vi "all_subvis.vi"   [LabVIEW 8.6]
uses:
  Controls/lxw_alignment.ctl
  Controls/lxw_boolean.ctl
  Controls/lxw_border_style.ctl
  Controls/lxw_chart_axis_label_position.ctl
  Controls/lxw_chart_axis_type.ctl
  Controls/lxw_chart_legend_position.ctl
  Controls/lxw_chart_marker_type.ctl
  Controls/lxw_chart_type.ctl
  Controls/lxw_defined_colors.ctl
  Controls/lxw_error.ctl
  Controls/lxw_filter_criteria.ctl
  Controls/lxw_filter_operator.ctl
  Controls/lxw_filter_rule.ctl
  Controls/lxw_pattern_type.ctl
  Controls/style_id.ctl
types:
  T1 = typedef "style_id.ctl" = u16
  T2 = typedef "lxw_pattern_type.ctl" = u8
  T3 = typedef "lxw_filter_rule.ctl" = cluster{"criteria":T4, "value_string":string, "value":dbl}
  T4 = typedef "lxw_filter_criteria.ctl" = u32
  T5 = typedef "lxw_filter_operator.ctl" = u8
  T6 = typedef "lxw_error.ctl" = u32
  T7 = typedef "lxw_defined_colors.ctl" = u32
  T8 = typedef "lxw_chart_type.ctl" = u8
  T9 = typedef "lxw_chart_marker_type.ctl" = u8
  T10 = typedef "lxw_chart_legend_position.ctl" = u8
  T11 = typedef "lxw_chart_axis_type.ctl" = u8
  T12 = typedef "lxw_chart_axis_label_position.ctl" = u8
  T13 = typedef "lxw_border_style.ctl" = u8
  T14 = typedef "lxw_boolean.ctl" = u8
  T15 = typedef "lxw_alignment.ctl" = u8
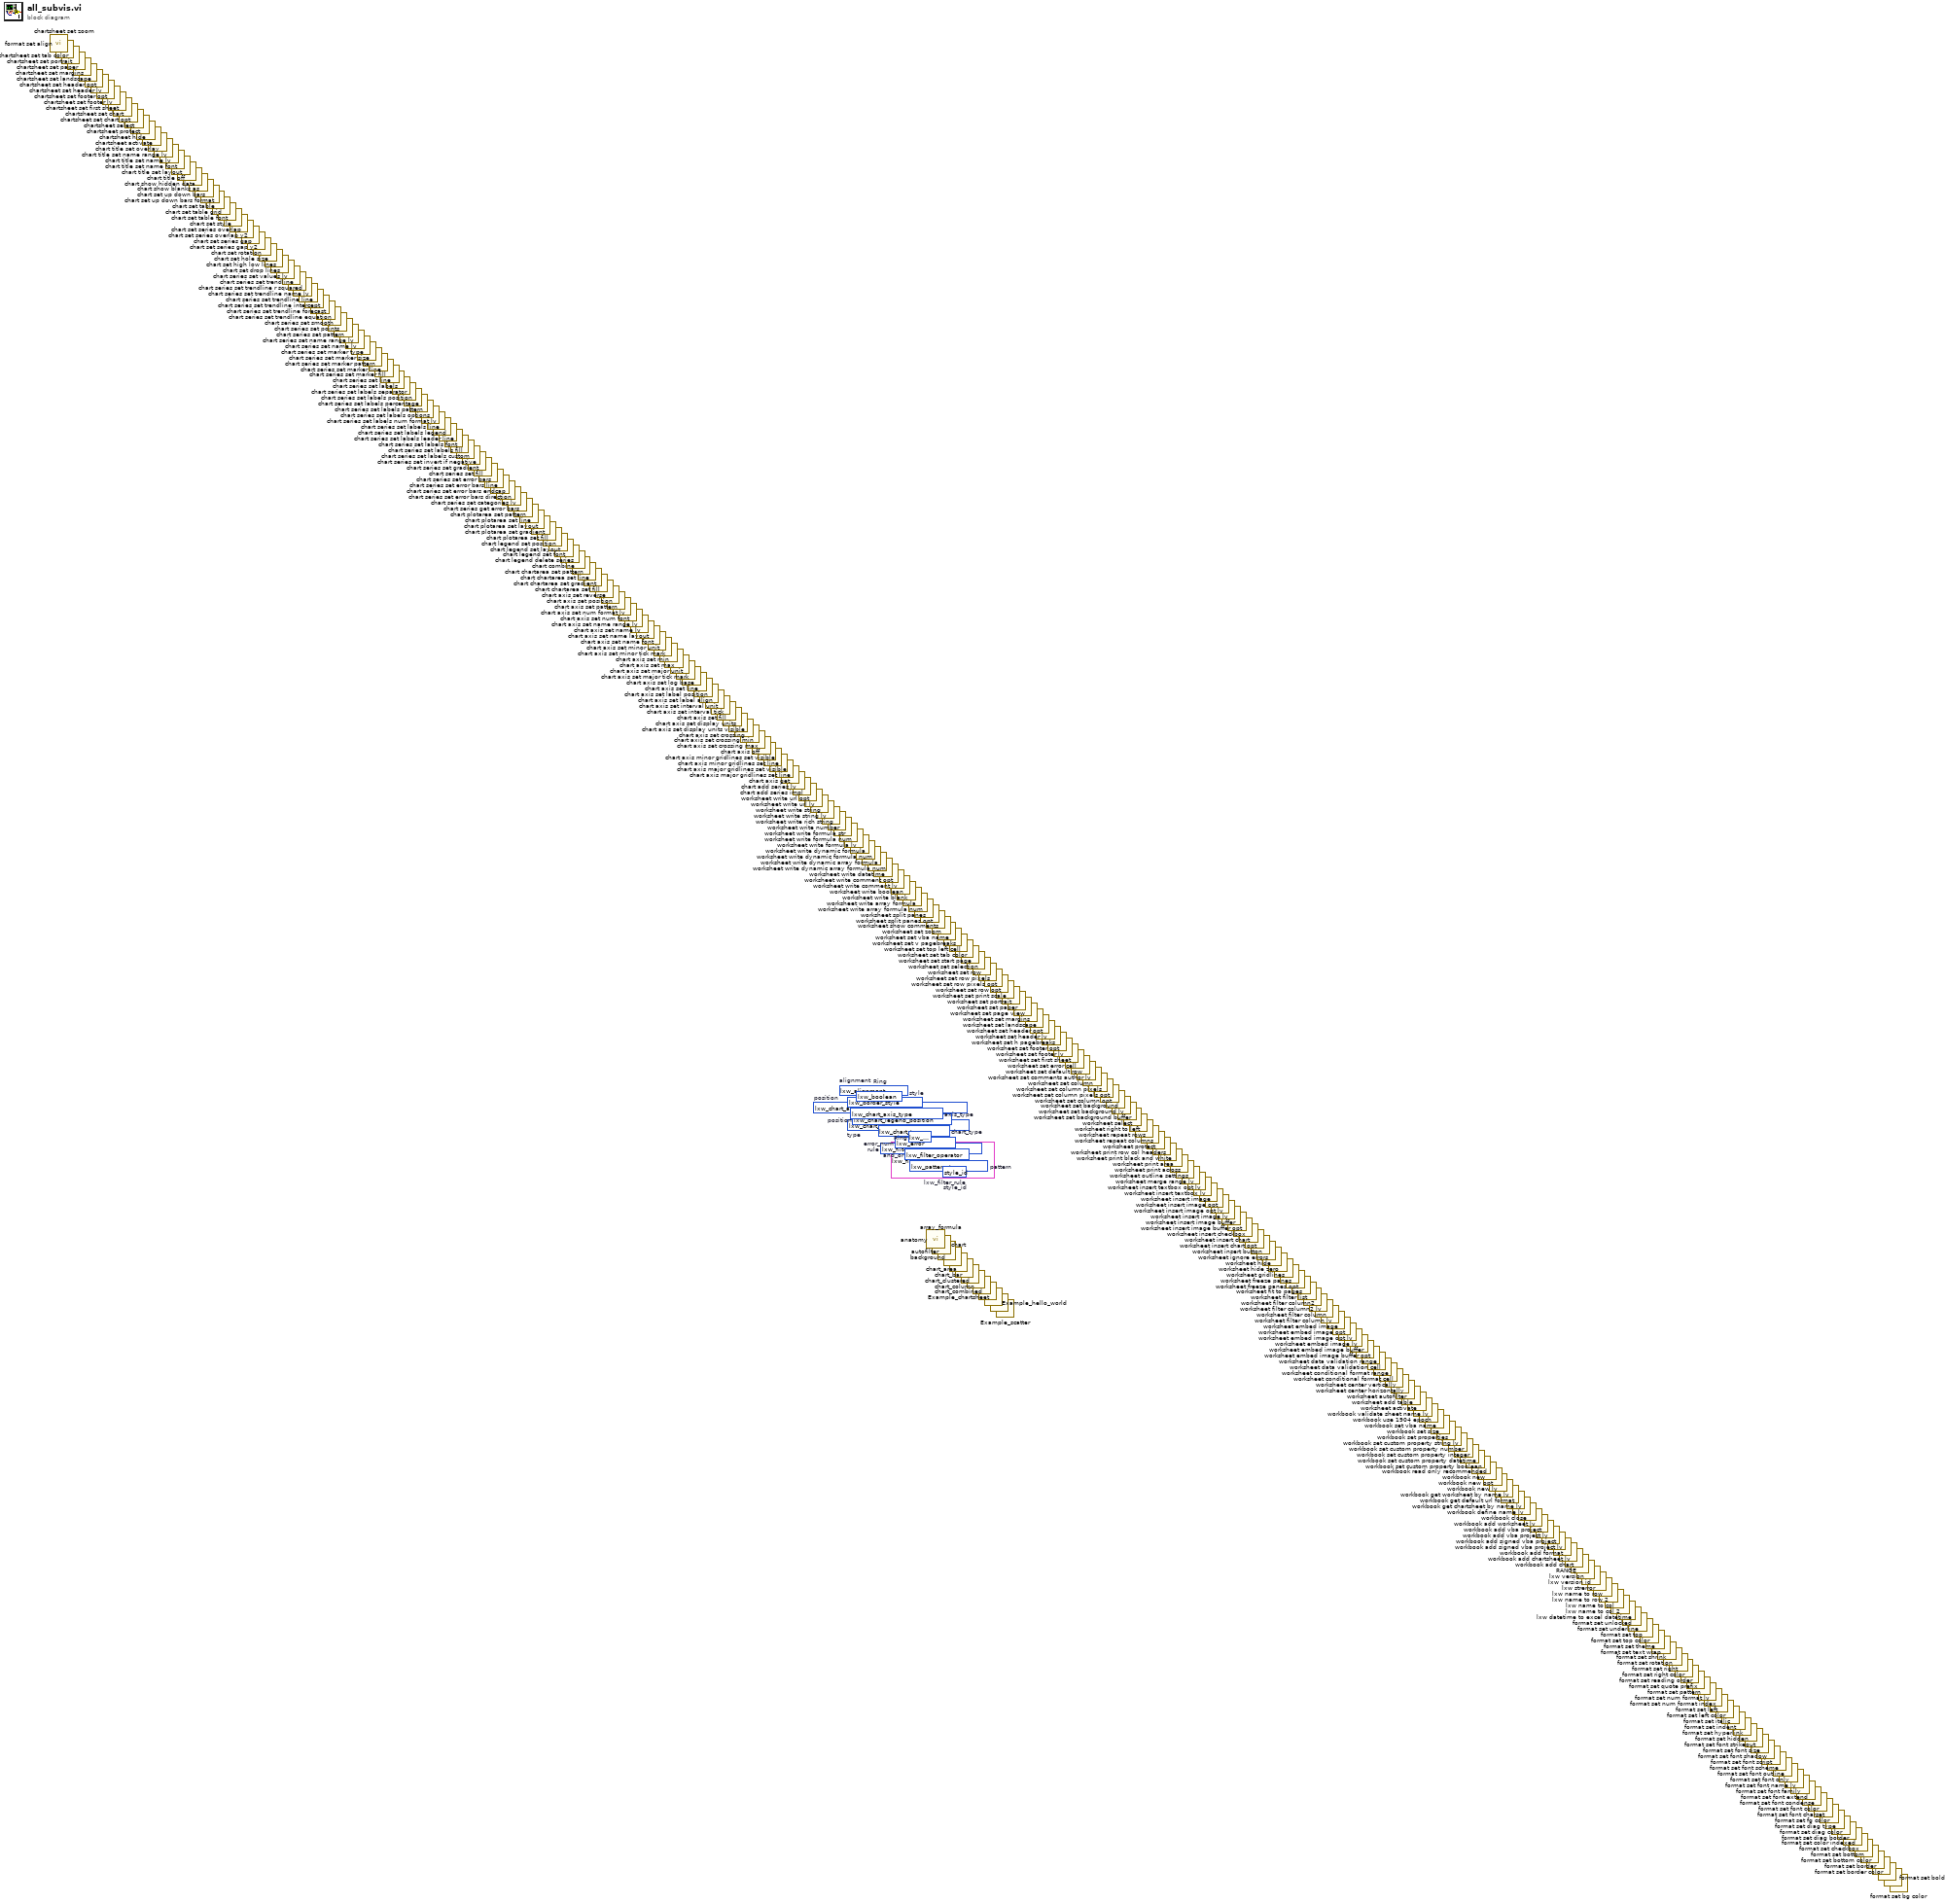
[diagram p0: block diagram]
diagram:
  (unwired) T1 ? items=["Style_1", "Style_2", "Style_3", "Style_4", "Style_5", "Style_6", "Style_7", "Style_8", "Style_9", "Style_10", "Style_11", "Style_12", "Style_13", "Style_14", "Style_15", "Style_16", "Style_17", "Style_18", "Style_19", "Style_20", "Style_21", "Style_22", "Style_23", "Style_24", "Style_25", "Style_26", "Style_27", "Style_28", "Style_29", "Style_30", "Style_31", "Style_32", "Style_33", "Style_34", "Style_35", "Style_36", "Style_37", "Style_38", "Style_39", "Style_40", "Style_41", "Style_42", "Style_43", "Style_44", "Style_45", "Style_46", "Style_47", "Style_48"]  # style_id
  (unwired) T2 ? items=["LXW_PATTERN_NONE", "LXW_PATTERN_SOLID", "LXW_PATTERN_MEDIUM_GRAY", "LXW_PATTERN_DARK_GRAY", "LXW_PATTERN_LIGHT_GRAY"]  # pattern
  (unwired) T3 ?  # lxw_filter_rule
  (unwired) T5 ? items=["LXW_FILTER_AND", "LXW_FILTER_OR"]  # and_or
  (unwired) T4 ? items=["LXW_FILTER_CRITERIA_NONE", "LXW_FILTER_CRITERIA_EQUAL_TO", "LXW_FILTER_CRITERIA_NOT_EQUAL_TO", "LXW_FILTER_CRITERIA_GREATER_THAN", "LXW_FILTER_CRITERIA_LESS_THAN", "LXW_FILTER_CRITERIA_GREATER_THAN_OR_EQUAL_TO", "LXW_FILTER_CRITERIA_LESS_THAN_OR_EQUAL_TO", "LXW_FILTER_CRITERIA_BLANKS", "LXW_FILTER_CRITERIA_NON_BLANKS"]  # rule
  (unwired) T6 ? items=["LXW_NO_ERROR", "LXW_ERROR_MEMORY_MALLOC_FAILED", "LXW_ERROR_CREATING_XLSX_FILE", "LXW_ERROR_CREATING_TMPFILE", "LXW_ERROR_READING_TMPFILE", "LXW_ERROR_ZIP_FILE_OPERATION", "LXW_ERROR_ZIP_PARAMETER_ERROR", "LXW_ERROR_ZIP_BAD_ZIP_FILE", "LXW_ERROR_ZIP_INTERNAL_ERROR", "LXW_ERROR_ZIP_FILE_ADD", "LXW_ERROR_ZIP_CLOSE", "LXW_ERROR_FEATURE_NOT_SUPPORTED", "LXW_ERROR_NULL_PARAMETER_IGNORED", "LXW_ERROR_PARAMETER_VALIDATION", "LXW_ERROR_WORKSHEET_INDEX_OUT_OF_RANGE"]  # error_num
  (unwired) T7 ? items=["LXW_COLOR_BLACK", "LXW_COLOR_BLUE", "LXW_COLOR_BROWN", "LXW_COLOR_CYAN", "LXW_COLOR_GRAY", "LXW_COLOR_GREEN", "LXW_COLOR_LIME", "LXW_COLOR_MAGENTA", "LXW_COLOR_NAVY", "LXW_COLOR_ORANGE", "LXW_COLOR_PURPLE", "LXW_COLOR_RED", "LXW_COLOR_SILVER", "LXW_COLOR_WHITE", "LXW_COLOR_YELLOW"]  # Ring
  (unwired) T8 ? items=["LXW_CHART_NONE", "LXW_CHART_AREA", "LXW_CHART_AREA_STACKED", "LXW_CHART_AREA_STACKED_PERCENT", "LXW_CHART_BAR", "LXW_CHART_BAR_STACKED", "LXW_CHART_BAR_STACKED_PERCENT", "LXW_CHART_COLUMN", "LXW_CHART_COLUMN_STACKED", "LXW_CHART_COLUMN_STACKED_PERCENT", "LXW_CHART_DOUGHNUT", "LXW_CHART_LINE", "LXW_CHART_LINE_STACKED", "LXW_CHART_LINE_STACKED_PERCENT", "LXW_CHART_PIE", "LXW_CHART_SCATTER", "LXW_CHART_SCATTER_STRAIGHT", "LXW_CHART_SCATTER_STRAIGHT_WITH_MARKERS", "LXW_CHART_SCATTER_SMOOTH", "LXW_CHART_SCATTER_SMOOTH_WITH_MARKERS", "LXW_CHART_RADAR", "LXW_CHART_RADAR_WITH_MARKERS", "LXW_CHART_RADAR_FILLED", "LXW_CHART_STOCK"]  # chart_type
  (unwired) T9 ? items=["LXW_CHART_MARKER_AUTOMATIC", "LXW_CHART_MARKER_NONE", "LXW_CHART_MARKER_SQUARE", "LXW_CHART_MARKER_DIAMOND", "LXW_CHART_MARKER_TRIANGLE", "LXW_CHART_MARKER_X", "LXW_CHART_MARKER_STAR", "LXW_CHART_MARKER_SHORT_DASH", "LXW_CHART_MARKER_LONG_DASH", "LXW_CHART_MARKER_CIRCLE", "LXW_CHART_MARKER_PLUS"]  # type
  (unwired) T10 ? items=["LXW_CHART_LEGEND_NONE", "LXW_CHART_LEGEND_RIGHT", "LXW_CHART_LEGEND_LEFT", "LXW_CHART_LEGEND_TOP", "LXW_CHART_LEGEND_BOTTOM", "LXW_CHART_LEGEND_TOP_RIGHT", "LXW_CHART_LEGEND_OVERLAY_RIGHT", "LXW_CHART_LEGEND_OVERLAY_LEFT"]  # position
  (unwired) T11 ? items=["LXW_CHART_AXIS_TYPE_X", "LXW_CHART_AXIS_TYPE_Y", "LXW_CHART_AXIS_TYPE_X2", "LXW_CHART_AXIS_TYPE_Y2"]  # axis_type
  (unwired) T12 ? items=["LXW_CHART_AXIS_LABEL_POSITION_NEXT_TO", "LXW_CHART_AXIS_LABEL_POSITION_HIGH", "LXW_CHART_AXIS_LABEL_POSITION_LOW", "LXW_CHART_AXIS_LABEL_POSITION_NONE"]  # position
  (unwired) T13 ? items=["LXW_BORDER_NONE", "LXW_BORDER_THIN", "LXW_BORDER_MEDIUM", "LXW_BORDER_DASHED", "LXW_BORDER_DOTTED", "LXW_BORDER_THICK", "LXW_BORDER_DOUBLE", "LXW_BORDER_HAIR"]  # style
  (unwired) T14 ? items=["LXW_FALSE", "LXW_TRUE", "LXW_EXPLICIT_FALSE"]  # Ring
  (unwired) T15 ? items=["LXW_ALIGN_NONE", "LXW_ALIGN_LEFT", "LXW_ALIGN_CENTER", "LXW_ALIGN_RIGHT", "LXW_ALIGN_FILL", "LXW_ALIGN_JUSTIFY", "LXW_ALIGN_CENTER_ACROSS", "LXW_ALIGN_DISTRIBUTED", "LXW_ALIGN_VERTICAL_TOP", "LXW_ALIGN_VERTICAL_BOTTOM", "LXW_ALIGN_VERTICAL_CENTER", "LXW_ALIGN_VERTICAL_JUSTIFY", "LXW_ALIGN_VERTICAL_DISTRIBUTED"]  # alignment
  n1 = call "format set align.vi"() -> ()  [unwired: 11 in, 1 out]
  n2 = call "chartsheet set zoom.vi"() -> ()  [unwired: 11 in, 1 out]
  n3 = call "chartsheet set tab color.vi"() -> ()  [unwired: 11 in, 1 out]
  n4 = call "chartsheet set portrait.vi"() -> ()  [unwired: 11 in, 1 out]
  n5 = call "chartsheet set paper.vi"() -> ()  [unwired: 11 in, 1 out]
  n6 = call "chartsheet set margins.vi"() -> ()  [unwired: 11 in, 1 out]
  n7 = call "chartsheet set landscape.vi"() -> ()  [unwired: 11 in, 1 out]
  n8 = call "chartsheet set header opt.vi"() -> ()  [unwired: 9 in, 3 out]
  n9 = call "chartsheet set header lv.vi"() -> ()  [unwired: 10 in, 2 out]
  n10 = call "chartsheet set footer opt.vi"() -> ()  [unwired: 9 in, 3 out]
  n11 = call "chartsheet set footer lv.vi"() -> ()  [unwired: 10 in, 2 out]
  n12 = call "chartsheet set first sheet.vi"() -> ()  [unwired: 11 in, 1 out]
  n13 = call "chartsheet set chart.vi"() -> ()  [unwired: 10 in, 2 out]
  n14 = call "chartsheet set chart opt.vi"() -> ()  [unwired: 9 in, 3 out]
  n15 = call "chartsheet select.vi"() -> ()  [unwired: 11 in, 1 out]
  n16 = call "chartsheet protect.vi"() -> ()  [unwired: 10 in, 2 out]
  n17 = call "chartsheet hide.vi"() -> ()  [unwired: 11 in, 1 out]
  n18 = call "chartsheet activate.vi"() -> ()  [unwired: 11 in, 1 out]
  n19 = call "chart title set overlay.vi"() -> ()  [unwired: 11 in, 1 out]
  n20 = call "chart title set name range lv.vi"() -> ()  [unwired: 11 in, 1 out]
  n21 = call "chart title set name lv.vi"() -> ()  [unwired: 11 in, 1 out]
  n22 = call "chart title set name font.vi"() -> ()  [unwired: 10 in, 2 out]
  n23 = call "chart title set layout.vi"() -> ()  [unwired: 10 in, 2 out]
  n24 = call "chart title off.vi"() -> ()  [unwired: 11 in, 1 out]
  n25 = call "chart show hidden data.vi"() -> ()  [unwired: 11 in, 1 out]
  n26 = call "chart show blanks as.vi"() -> ()  [unwired: 11 in, 1 out]
  n27 = call "chart set up down bars.vi"() -> ()  [unwired: 11 in, 1 out]
  n28 = call "chart set up down bars format.vi"() -> ()  [unwired: 11 in, 5 out]
  n29 = call "chart set table.vi"() -> ()  [unwired: 11 in, 1 out]
  n30 = call "chart set table grid.vi"() -> ()  [unwired: 11 in, 1 out]
  n31 = call "chart set table font.vi"() -> ()  [unwired: 10 in, 2 out]
  n32 = call "chart set style.vi"() -> ()  [unwired: 11 in, 1 out]
  n33 = call "chart set series overlap.vi"() -> ()  [unwired: 11 in, 1 out]
  n34 = call "chart set series overlap y2.vi"() -> ()  [unwired: 11 in, 1 out]
  n35 = call "chart set series gap.vi"() -> ()  [unwired: 11 in, 1 out]
  n36 = call "chart set series gap y2.vi"() -> ()  [unwired: 11 in, 1 out]
  n37 = call "chart set rotation.vi"() -> ()  [unwired: 11 in, 1 out]
  n38 = call "chart set hole size.vi"() -> ()  [unwired: 11 in, 1 out]
  n39 = call "chart set high low lines.vi"() -> ()  [unwired: 10 in, 2 out]
  n40 = call "chart set drop lines.vi"() -> ()  [unwired: 10 in, 2 out]
  n41 = call "chart series set values lv.vi"() -> ()  [unwired: 11 in, 1 out]
  n42 = call "chart series set trendline.vi"() -> ()  [unwired: 11 in, 1 out]
  n43 = call "chart series set trendline r squared.vi"() -> ()  [unwired: 11 in, 1 out]
  n44 = call "chart series set trendline name lv.vi"() -> ()  [unwired: 11 in, 1 out]
  n45 = call "chart series set trendline line.vi"() -> ()  [unwired: 10 in, 2 out]
  n46 = call "chart series set trendline intercept.vi"() -> ()  [unwired: 11 in, 1 out]
  n47 = call "chart series set trendline forecast.vi"() -> ()  [unwired: 11 in, 1 out]
  n48 = call "chart series set trendline equation.vi"() -> ()  [unwired: 11 in, 1 out]
  n49 = call "chart series set smooth.vi"() -> ()  [unwired: 11 in, 1 out]
  n50 = call "chart series set points.vi"() -> ()  [unwired: 10 in, 2 out]
  n51 = call "chart series set pattern.vi"() -> ()  [unwired: 10 in, 2 out]
  n52 = call "chart series set name range lv.vi"() -> ()  [unwired: 11 in, 1 out]
  n53 = call "chart series set name lv.vi"() -> ()  [unwired: 11 in, 1 out]
  n54 = call "chart series set marker type.vi"() -> ()  [unwired: 11 in, 1 out]
  n55 = call "chart series set marker size.vi"() -> ()  [unwired: 11 in, 1 out]
  n56 = call "chart series set marker pattern.vi"() -> ()  [unwired: 10 in, 2 out]
  n57 = call "chart series set marker line.vi"() -> ()  [unwired: 10 in, 2 out]
  n58 = call "chart series set marker fill.vi"() -> ()  [unwired: 10 in, 2 out]
  n59 = call "chart series set line.vi"() -> ()  [unwired: 10 in, 2 out]
  n60 = call "chart series set labels.vi"() -> ()  [unwired: 11 in, 1 out]
  n61 = call "chart series set labels separator.vi"() -> ()  [unwired: 11 in, 1 out]
  n62 = call "chart series set labels position.vi"() -> ()  [unwired: 11 in, 1 out]
  n63 = call "chart series set labels percentage.vi"() -> ()  [unwired: 11 in, 1 out]
  n64 = call "chart series set labels pattern.vi"() -> ()  [unwired: 10 in, 2 out]
  n65 = call "chart series set labels options.vi"() -> ()  [unwired: 11 in, 1 out]
  n66 = call "chart series set labels num format lv.vi"() -> ()  [unwired: 11 in, 1 out]
  n67 = call "chart series set labels line.vi"() -> ()  [unwired: 10 in, 2 out]
  n68 = call "chart series set labels legend.vi"() -> ()  [unwired: 11 in, 1 out]
  n69 = call "chart series set labels leader line.vi"() -> ()  [unwired: 11 in, 1 out]
  n70 = call "chart series set labels font.vi"() -> ()  [unwired: 10 in, 2 out]
  n71 = call "chart series set labels fill.vi"() -> ()  [unwired: 10 in, 2 out]
  n72 = call "chart series set labels custom.vi"() -> ()  [unwired: 10 in, 2 out]
  n73 = call "chart series set invert if negative.vi"() -> ()  [unwired: 11 in, 1 out]
  n74 = call "chart series set gradient.vi"() -> ()  [unwired: 10 in, 2 out]
  n75 = call "chart series set fill.vi"() -> ()  [unwired: 10 in, 2 out]
  n76 = call "chart series set error bars.vi"() -> ()  [unwired: 11 in, 1 out]
  n77 = call "chart series set error bars line.vi"() -> ()  [unwired: 10 in, 2 out]
  n78 = call "chart series set error bars endcap.vi"() -> ()  [unwired: 11 in, 1 out]
  n79 = call "chart series set error bars direction.vi"() -> ()  [unwired: 11 in, 1 out]
  n80 = call "chart series set categories lv.vi"() -> ()  [unwired: 11 in, 1 out]
  n81 = call "chart series get error bars.vi"() -> ()  [unwired: 10 in, 2 out]
  n82 = call "chart plotarea set pattern.vi"() -> ()  [unwired: 10 in, 2 out]
  n83 = call "chart plotarea set line.vi"() -> ()  [unwired: 10 in, 2 out]
  n84 = call "chart plotarea set layout.vi"() -> ()  [unwired: 10 in, 2 out]
  n85 = call "chart plotarea set gradient.vi"() -> ()  [unwired: 10 in, 2 out]
  n86 = call "chart plotarea set fill.vi"() -> ()  [unwired: 10 in, 2 out]
  n87 = call "chart legend set position.vi"() -> ()  [unwired: 11 in, 1 out]
  n88 = call "chart legend set layout.vi"() -> ()  [unwired: 10 in, 2 out]
  n89 = call "chart legend set font.vi"() -> ()  [unwired: 10 in, 2 out]
  n90 = call "chart legend delete series.vi"() -> ()  [unwired: 10 in, 2 out]
  n91 = call "chart combine.vi"() -> ()  [unwired: 11 in, 1 out]
  n92 = call "chart chartarea set pattern.vi"() -> ()  [unwired: 10 in, 2 out]
  n93 = call "chart chartarea set line.vi"() -> ()  [unwired: 10 in, 2 out]
  n94 = call "chart chartarea set gradient.vi"() -> ()  [unwired: 10 in, 2 out]
  n95 = call "chart chartarea set fill.vi"() -> ()  [unwired: 10 in, 2 out]
  n96 = call "chart axis set reverse.vi"() -> ()  [unwired: 11 in, 1 out]
  n97 = call "chart axis set position.vi"() -> ()  [unwired: 11 in, 1 out]
  n98 = call "chart axis set pattern.vi"() -> ()  [unwired: 10 in, 2 out]
  n99 = call "chart axis set num format lv.vi"() -> ()  [unwired: 11 in, 1 out]
  n100 = call "chart axis set num font.vi"() -> ()  [unwired: 10 in, 2 out]
  n101 = call "chart axis set name range lv.vi"() -> ()  [unwired: 11 in, 1 out]
  n102 = call "chart axis set name lv.vi"() -> ()  [unwired: 11 in, 1 out]
  n103 = call "chart axis set name layout.vi"() -> ()  [unwired: 10 in, 2 out]
  n104 = call "chart axis set name font.vi"() -> ()  [unwired: 10 in, 2 out]
  n105 = call "chart axis set minor unit.vi"() -> ()  [unwired: 11 in, 1 out]
  n106 = call "chart axis set minor tick mark.vi"() -> ()  [unwired: 11 in, 1 out]
  n107 = call "chart axis set min.vi"() -> ()  [unwired: 11 in, 1 out]
  n108 = call "chart axis set max.vi"() -> ()  [unwired: 11 in, 1 out]
  n109 = call "chart axis set major unit.vi"() -> ()  [unwired: 11 in, 1 out]
  n110 = call "chart axis set major tick mark.vi"() -> ()  [unwired: 11 in, 1 out]
  n111 = call "chart axis set log base.vi"() -> ()  [unwired: 11 in, 1 out]
  n112 = call "chart axis set line.vi"() -> ()  [unwired: 10 in, 2 out]
  n113 = call "chart axis set label position.vi"() -> ()  [unwired: 11 in, 1 out]
  n114 = call "chart axis set label align.vi"() -> ()  [unwired: 11 in, 1 out]
  n115 = call "chart axis set interval unit.vi"() -> ()  [unwired: 11 in, 1 out]
  n116 = call "chart axis set interval tick.vi"() -> ()  [unwired: 11 in, 1 out]
  n117 = call "chart axis set fill.vi"() -> ()  [unwired: 10 in, 2 out]
  n118 = call "chart axis set display units.vi"() -> ()  [unwired: 11 in, 1 out]
  n119 = call "chart axis set display units visible.vi"() -> ()  [unwired: 11 in, 1 out]
  n120 = call "chart axis set crossing.vi"() -> ()  [unwired: 11 in, 1 out]
  n121 = call "chart axis set crossing min.vi"() -> ()  [unwired: 11 in, 1 out]
  n122 = call "chart axis set crossing max.vi"() -> ()  [unwired: 11 in, 1 out]
  n123 = call "chart axis off.vi"() -> ()  [unwired: 11 in, 1 out]
  n124 = call "chart axis minor gridlines set visible.vi"() -> ()  [unwired: 11 in, 1 out]
  n125 = call "chart axis minor gridlines set line.vi"() -> ()  [unwired: 10 in, 2 out]
  n126 = call "chart axis major gridlines set visible.vi"() -> ()  [unwired: 11 in, 1 out]
  n127 = call "chart axis major gridlines set line.vi"() -> ()  [unwired: 10 in, 2 out]
  n128 = call "chart axis get.vi"() -> ()  [unwired: 10 in, 2 out]
  n129 = call "chart add series lv.vi"() -> ()  [unwired: 10 in, 2 out]
  n130 = call "chart add series impl.vi"() -> ()  [unwired: 10 in, 2 out]
  n131 = call "worksheet write url opt.vi"() -> ()  [unwired: 10 in, 2 out]
  n132 = call "worksheet write url lv.vi"() -> ()  [unwired: 10 in, 2 out]
  n133 = call "worksheet write string.vi"() -> ()  [unwired: 10 in, 2 out]
  n134 = call "worksheet write string lv.vi"() -> ()  [unwired: 10 in, 2 out]
  n135 = call "worksheet write rich string.vi"() -> ()  [unwired: 10 in, 2 out]
  n136 = call "worksheet write number.vi"() -> ()  [unwired: 10 in, 2 out]
  n137 = call "worksheet write formula str.vi"() -> ()  [unwired: 10 in, 2 out]
  n138 = call "worksheet write formula num.vi"() -> ()  [unwired: 10 in, 2 out]
  n139 = call "worksheet write formula lv.vi"() -> ()  [unwired: 10 in, 2 out]
  n140 = call "worksheet write dynamic formula.vi"() -> ()  [unwired: 10 in, 2 out]
  n141 = call "worksheet write dynamic formula num.vi"() -> ()  [unwired: 10 in, 2 out]
  n142 = call "worksheet write dynamic array formula.vi"() -> ()  [unwired: 10 in, 2 out]
  n143 = call "worksheet write dynamic array formula num.vi"() -> ()  [unwired: 14 in, 2 out]
  n144 = call "worksheet write datetime.vi"() -> ()  [unwired: 9 in, 3 out]
  n145 = call "worksheet write comment opt.vi"() -> ()  [unwired: 10 in, 2 out]
  n146 = call "worksheet write comment lv.vi"() -> ()  [unwired: 10 in, 2 out]
  n147 = call "worksheet write boolean.vi"() -> ()  [unwired: 10 in, 2 out]
  n148 = call "worksheet write blank.vi"() -> ()  [unwired: 10 in, 2 out]
  n149 = call "worksheet write array formula.vi"() -> ()  [unwired: 10 in, 2 out]
  n150 = call "worksheet write array formula num.vi"() -> ()  [unwired: 14 in, 2 out]
  n151 = call "worksheet split panes.vi"() -> ()  [unwired: 11 in, 1 out]
  n152 = call "worksheet split panes opt.vi"() -> ()  [unwired: 11 in, 1 out]
  n153 = call "anatomy.vi"() -> ()  [unwired: 12 in]
  n154 = call "worksheet show comments.vi"() -> ()  [unwired: 11 in, 1 out]
  n155 = call "array_formula.vi"() -> ()  [unwired: 12 in]
  n156 = call "worksheet set zoom.vi"() -> ()  [unwired: 11 in, 1 out]
  n157 = call "autofilter.vi"() -> ()  [unwired: 12 in]
  n158 = call "worksheet set vba name.vi"() -> ()  [unwired: 10 in, 2 out]
  n159 = call "background.vi"() -> ()  [unwired: 12 in]
  n160 = call "worksheet set v pagebreaks.vi"() -> ()  [unwired: 10 in, 2 out]
  n161 = call "chart.vi"() -> ()  [unwired: 12 in]
  n162 = call "worksheet set top left cell.vi"() -> ()  [unwired: 11 in, 1 out]
  n163 = call "chart_area.vi"() -> ()  [unwired: 12 in]
  n164 = call "worksheet set tab color.vi"() -> ()  [unwired: 11 in, 1 out]
  n165 = call "chart_bar.vi"() -> ()  [unwired: 12 in]
  n166 = call "worksheet set start page.vi"() -> ()  [unwired: 11 in, 1 out]
  n167 = call "chart_clustered.vi"() -> ()  [unwired: 12 in]
  n168 = call "worksheet set selection.vi"() -> ()  [unwired: 10 in, 2 out]
  n169 = call "chart_column.vi"() -> ()  [unwired: 12 in]
  n170 = call "worksheet set row.vi"() -> ()  [unwired: 10 in, 2 out]
  n171 = call "chart_combined.vi"() -> ()  [unwired: 12 in]
  n172 = call "worksheet set row pixels.vi"() -> ()  [unwired: 10 in, 2 out]
  n173 = call "Example_chartsheet.vi"() -> ()  [unwired: 12 in]
  n174 = call "worksheet set row pixels opt.vi"() -> ()  [unwired: 9 in, 3 out]
  n175 = call "Example_hello_world.vi"() -> ()  [unwired: 12 in]
  n176 = call "worksheet set row opt.vi"() -> ()  [unwired: 9 in, 3 out]
  n177 = call "Example_scatter.vi"() -> ()  [unwired: 12 in]
  n178 = call "worksheet set print scale.vi"() -> ()  [unwired: 11 in, 1 out]
  n179 = call "worksheet set portrait.vi"() -> ()  [unwired: 11 in, 1 out]
  n180 = call "worksheet set paper.vi"() -> ()  [unwired: 11 in, 1 out]
  n181 = call "worksheet set page view.vi"() -> ()  [unwired: 11 in, 1 out]
  n182 = call "worksheet set margins.vi"() -> ()  [unwired: 11 in, 1 out]
  n183 = call "worksheet set landscape.vi"() -> ()  [unwired: 11 in, 1 out]
  n184 = call "worksheet set header opt.vi"() -> ()  [unwired: 9 in, 3 out]
  n185 = call "worksheet set header lv.vi"() -> ()  [unwired: 10 in, 2 out]
  n186 = call "worksheet set h pagebreaks.vi"() -> ()  [unwired: 10 in, 2 out]
  n187 = call "worksheet set footer opt.vi"() -> ()  [unwired: 9 in, 3 out]
  n188 = call "worksheet set footer lv.vi"() -> ()  [unwired: 10 in, 2 out]
  n189 = call "worksheet set first sheet.vi"() -> ()  [unwired: 11 in, 1 out]
  n190 = call "worksheet set error cell.vi"() -> ()  [unwired: 11 in, 1 out]
  n191 = call "worksheet set default row.vi"() -> ()  [unwired: 11 in, 1 out]
  n192 = call "worksheet set comments author lv.vi"() -> ()  [unwired: 11 in, 1 out]
  n193 = call "worksheet set column.vi"() -> ()  [unwired: 10 in, 2 out]
  n194 = call "worksheet set column pixels.vi"() -> ()  [unwired: 10 in, 2 out]
  n195 = call "worksheet set column pixels opt.vi"() -> ()  [unwired: 9 in, 3 out]
  n196 = call "worksheet set column opt.vi"() -> ()  [unwired: 9 in, 3 out]
  n197 = call "worksheet set background.vi"() -> ()  [unwired: 10 in, 2 out]
  n198 = call "worksheet set background lv.vi"() -> ()  [unwired: 10 in, 2 out]
  n199 = call "worksheet set background buffer.vi"() -> ()  [unwired: 10 in, 2 out]
  n200 = call "worksheet select.vi"() -> ()  [unwired: 11 in, 1 out]
  n201 = call "worksheet right to left.vi"() -> ()  [unwired: 11 in, 1 out]
  n202 = call "worksheet repeat rows.vi"() -> ()  [unwired: 10 in, 2 out]
  n203 = call "worksheet repeat columns.vi"() -> ()  [unwired: 10 in, 2 out]
  n204 = call "worksheet protect.vi"() -> ()  [unwired: 10 in, 2 out]
  n205 = call "worksheet print row col headers.vi"() -> ()  [unwired: 11 in, 1 out]
  n206 = call "worksheet print black and white.vi"() -> ()  [unwired: 11 in, 1 out]
  n207 = call "worksheet print area.vi"() -> ()  [unwired: 10 in, 2 out]
  n208 = call "worksheet print across.vi"() -> ()  [unwired: 11 in, 1 out]
  n209 = call "worksheet outline settings.vi"() -> ()  [unwired: 11 in, 1 out]
  n210 = call "worksheet merge range lv.vi"() -> ()  [unwired: 10 in, 2 out]
  n211 = call "worksheet insert textbox opt lv.vi"() -> ()  [unwired: 9 in, 3 out]
  n212 = call "worksheet insert textbox lv.vi"() -> ()  [unwired: 10 in, 2 out]
  n213 = call "worksheet insert image.vi"() -> ()  [unwired: 10 in, 2 out]
  n214 = call "worksheet insert image opt.vi"() -> ()  [unwired: 9 in, 3 out]
  n215 = call "worksheet insert image opt lv.vi"() -> ()  [unwired: 9 in, 3 out]
  n216 = call "worksheet insert image lv.vi"() -> ()  [unwired: 10 in, 2 out]
  n217 = call "worksheet insert image buffer.vi"() -> ()  [unwired: 10 in, 2 out]
  n218 = call "worksheet insert image buffer opt.vi"() -> ()  [unwired: 9 in, 3 out]
  n219 = call "worksheet insert checkbox.vi"() -> ()  [unwired: 10 in, 2 out]
  n220 = call "worksheet insert chart.vi"() -> ()  [unwired: 10 in, 2 out]
  n221 = call "worksheet insert chart opt.vi"() -> ()  [unwired: 9 in, 3 out]
  n222 = call "worksheet insert button.vi"() -> ()  [unwired: 9 in, 3 out]
  n223 = call "worksheet ignore errors.vi"() -> ()  [unwired: 10 in, 2 out]
  n224 = call "worksheet hide.vi"() -> ()  [unwired: 11 in, 1 out]
  n225 = call "worksheet hide zero.vi"() -> ()  [unwired: 11 in, 1 out]
  n226 = call "worksheet gridlines.vi"() -> ()  [unwired: 11 in, 1 out]
  n227 = call "worksheet freeze panes.vi"() -> ()  [unwired: 11 in, 1 out]
  n228 = call "worksheet freeze panes opt.vi"() -> ()  [unwired: 11 in, 1 out]
  n229 = call "worksheet fit to pages.vi"() -> ()  [unwired: 11 in, 1 out]
  n230 = call "worksheet filter list.vi"() -> ()  [unwired: 10 in, 2 out]
  n231 = call "worksheet filter column2.vi"() -> ()  [unwired: 10 in, 2 out]
  n232 = call "worksheet filter column2 lv.vi"() -> ()  [unwired: 10 in, 2 out]
  n233 = call "worksheet filter column.vi"() -> ()  [unwired: 10 in, 2 out]
  n234 = call "worksheet filter column lv.vi"() -> ()  [unwired: 9 in, 3 out]
  n235 = call "worksheet embed image.vi"() -> ()  [unwired: 10 in, 2 out]
  n236 = call "worksheet embed image opt.vi"() -> ()  [unwired: 9 in, 3 out]
  n237 = call "worksheet embed image opt lv.vi"() -> ()  [unwired: 9 in, 3 out]
  n238 = call "worksheet embed image lv.vi"() -> ()  [unwired: 10 in, 2 out]
  n239 = call "worksheet embed image buffer.vi"() -> ()  [unwired: 10 in, 2 out]
  n240 = call "worksheet embed image buffer opt.vi"() -> ()  [unwired: 9 in, 3 out]
  n241 = call "worksheet data validation range.vi"() -> ()  [unwired: 10 in, 2 out]
  n242 = call "worksheet data validation cell.vi"() -> ()  [unwired: 10 in, 2 out]
  n243 = call "worksheet conditional format range.vi"() -> ()  [unwired: 10 in, 2 out]
  n244 = call "worksheet conditional format cell.vi"() -> ()  [unwired: 10 in, 2 out]
  n245 = call "worksheet center vertically.vi"() -> ()  [unwired: 11 in, 1 out]
  n246 = call "worksheet center horizontally.vi"() -> ()  [unwired: 11 in, 1 out]
  n247 = call "worksheet autofilter.vi"() -> ()  [unwired: 10 in, 2 out]
  n248 = call "worksheet add table.vi"() -> ()  [unwired: 10 in, 2 out]
  n249 = call "worksheet activate.vi"() -> ()  [unwired: 11 in, 1 out]
  n250 = call "workbook validate sheet name lv.vi"() -> ()  [unwired: 10 in, 2 out]
  n251 = call "workbook use 1904 epoch.vi"() -> ()  [unwired: 11 in, 1 out]
  n252 = call "workbook set vba name.vi"() -> ()  [unwired: 10 in, 2 out]
  n253 = call "workbook set size.vi"() -> ()  [unwired: 11 in, 1 out]
  n254 = call "workbook set properties.vi"() -> ()  [unwired: 10 in, 2 out]
  n255 = call "workbook set custom property string lv.vi"() -> ()  [unwired: 10 in, 2 out]
  n256 = call "workbook set custom property number.vi"() -> ()  [unwired: 10 in, 2 out]
  n257 = call "workbook set custom property integer.vi"() -> ()  [unwired: 10 in, 2 out]
  n258 = call "workbook set custom property datetime.vi"() -> ()  [unwired: 9 in, 3 out]
  n259 = call "workbook set custom property boolean.vi"() -> ()  [unwired: 10 in, 2 out]
  n260 = call "workbook read only recommended.vi"() -> ()  [unwired: 11 in, 1 out]
  n261 = call "workbook new.vi"() -> ()  [unwired: 10 in, 2 out]
  n262 = call "workbook new opt.vi"() -> ()  [unwired: 10 in, 2 out]
  n263 = call "workbook new lv.vi"() -> ()  [unwired: 10 in, 2 out]
  n264 = call "workbook get worksheet by name lv.vi"() -> ()  [unwired: 10 in, 2 out]
  n265 = call "workbook get default url format.vi"() -> ()  [unwired: 10 in, 2 out]
  n266 = call "workbook get chartsheet by name lv.vi"() -> ()  [unwired: 10 in, 2 out]
  n267 = call "workbook define name lv.vi"() -> ()  [unwired: 10 in, 2 out]
  n268 = call "workbook close.vi"() -> ()  [unwired: 10 in, 2 out]
  n269 = call "workbook add worksheet lv.vi"() -> ()  [unwired: 10 in, 2 out]
  n270 = call "workbook add vba project.vi"() -> ()  [unwired: 10 in, 2 out]
  n271 = call "workbook add vba project lv.vi"() -> ()  [unwired: 10 in, 2 out]
  n272 = call "workbook add signed vba project.vi"() -> ()  [unwired: 10 in, 2 out]
  n273 = call "workbook add signed vba project lv.vi"() -> ()  [unwired: 10 in, 2 out]
  n274 = call "workbook add format.vi"() -> ()  [unwired: 10 in, 2 out]
  n275 = call "workbook add chartsheet lv.vi"() -> ()  [unwired: 10 in, 2 out]
  n276 = call "workbook add chart.vi"() -> ()  [unwired: 10 in, 2 out]
  n277 = call "RANGE.vi"() -> ()  [unwired: 7 in, 5 out]
  n278 = call "lxw version.vi"() -> ()  [unwired: 10 in, 2 out]
  n279 = call "lxw version id.vi"() -> ()  [unwired: 10 in, 2 out]
  n280 = call "lxw strerror.vi"() -> ()  [unwired: 10 in, 2 out]
  n281 = call "lxw name to row.vi"() -> ()  [unwired: 10 in, 2 out]
  n282 = call "lxw name to row 2.vi"() -> ()  [unwired: 10 in, 2 out]
  n283 = call "lxw name to col.vi"() -> ()  [unwired: 10 in, 2 out]
  n284 = call "lxw name to col 2.vi"() -> ()  [unwired: 10 in, 2 out]
  n285 = call "lxw datetime to excel datetime.vi"() -> ()  [unwired: 9 in, 3 out]
  n286 = call "format set unlocked.vi"() -> ()  [unwired: 11 in, 1 out]
  n287 = call "format set underline.vi"() -> ()  [unwired: 11 in, 1 out]
  n288 = call "format set top.vi"() -> ()  [unwired: 11 in, 1 out]
  n289 = call "format set top color.vi"() -> ()  [unwired: 11 in, 1 out]
  n290 = call "format set theme.vi"() -> ()  [unwired: 11 in, 1 out]
  n291 = call "format set text wrap.vi"() -> ()  [unwired: 11 in, 1 out]
  n292 = call "format set shrink.vi"() -> ()  [unwired: 11 in, 1 out]
  n293 = call "format set rotation.vi"() -> ()  [unwired: 11 in, 1 out]
  n294 = call "format set right.vi"() -> ()  [unwired: 11 in, 1 out]
  n295 = call "format set right color.vi"() -> ()  [unwired: 11 in, 1 out]
  n296 = call "format set reading order.vi"() -> ()  [unwired: 11 in, 1 out]
  n297 = call "format set quote prefix.vi"() -> ()  [unwired: 11 in, 1 out]
  n298 = call "format set pattern.vi"() -> ()  [unwired: 11 in, 1 out]
  n299 = call "format set num format lv.vi"() -> ()  [unwired: 11 in, 1 out]
  n300 = call "format set num format index.vi"() -> ()  [unwired: 11 in, 1 out]
  n301 = call "format set left.vi"() -> ()  [unwired: 11 in, 1 out]
  n302 = call "format set left color.vi"() -> ()  [unwired: 11 in, 1 out]
  n303 = call "format set italic.vi"() -> ()  [unwired: 11 in, 1 out]
  n304 = call "format set indent.vi"() -> ()  [unwired: 11 in, 1 out]
  n305 = call "format set hyperlink.vi"() -> ()  [unwired: 11 in, 1 out]
  n306 = call "format set hidden.vi"() -> ()  [unwired: 11 in, 1 out]
  n307 = call "format set font strikeout.vi"() -> ()  [unwired: 11 in, 1 out]
  n308 = call "format set font size.vi"() -> ()  [unwired: 11 in, 1 out]
  n309 = call "format set font shadow.vi"() -> ()  [unwired: 11 in, 1 out]
  n310 = call "format set font script.vi"() -> ()  [unwired: 11 in, 1 out]
  n311 = call "format set font scheme.vi"() -> ()  [unwired: 11 in, 1 out]
  n312 = call "format set font outline.vi"() -> ()  [unwired: 11 in, 1 out]
  n313 = call "format set font only.vi"() -> ()  [unwired: 11 in, 1 out]
  n314 = call "format set font name lv.vi"() -> ()  [unwired: 11 in, 1 out]
  n315 = call "format set font family.vi"() -> ()  [unwired: 11 in, 1 out]
  n316 = call "format set font extend.vi"() -> ()  [unwired: 11 in, 1 out]
  n317 = call "format set font condense.vi"() -> ()  [unwired: 11 in, 1 out]
  n318 = call "format set font color.vi"() -> ()  [unwired: 11 in, 1 out]
  n319 = call "format set font charset.vi"() -> ()  [unwired: 11 in, 1 out]
  n320 = call "format set fg color.vi"() -> ()  [unwired: 11 in, 1 out]
  n321 = call "format set diag type.vi"() -> ()  [unwired: 11 in, 1 out]
  n322 = call "format set diag color.vi"() -> ()  [unwired: 11 in, 1 out]
  n323 = call "format set diag border.vi"() -> ()  [unwired: 11 in, 1 out]
  n324 = call "format set color indexed.vi"() -> ()  [unwired: 11 in, 1 out]
  n325 = call "format set checkbox.vi"() -> ()  [unwired: 11 in, 1 out]
  n326 = call "format set bottom.vi"() -> ()  [unwired: 11 in, 1 out]
  n327 = call "format set bottom color.vi"() -> ()  [unwired: 11 in, 1 out]
  n328 = call "format set border.vi"() -> ()  [unwired: 11 in, 1 out]
  n329 = call "format set border color.vi"() -> ()  [unwired: 11 in, 1 out]
  n330 = call "format set bold.vi"() -> ()  [unwired: 11 in, 1 out]
  n331 = call "format set bg color.vi"() -> ()  [unwired: 11 in, 1 out]
